vi "GetInfo.vi"(8 "error in (no error)":errorcluster, 10 "Parameter":variant, 11 "NiPxi6683H in":refnum<class "NiPxi6683H.lvclass">) -> (0 "error out":errorcluster, 2 "Info":string[](array[string]), 3 "NiPxi6683H out":refnum<class "NiPxi6683H.lvclass">)   [LabVIEW 2014, in "SyncPlugins.lvlib" / "NiPxi6683H.lvclass"]
uses:
  NiPxi6683H.lvclass
  NiPxi6682/NiPxi6682.lvclass/NiPxi6682.ctl
  NiPxi6683H.lvclass/NiPxi6683H.ctl
  NiPxi6682/Accessors/Read NiSyncHandle.vi
  Accessors/Read Triggers.vi
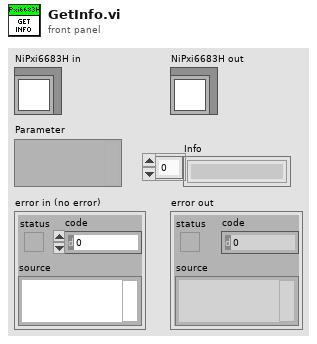
[diagram p1: front panel]
types:
  T1 = typedef "SyncPlugins.lvlib/PXI_MultiTrig.lvclass/clTrigger.ctl" = cluster{"Name":string, "DestTerm":string, "SrcTerm":string, "SyncClk":string, "Edge":i32, "Invert?":i32, "Initiated":bool, "Type":string, "TrigTime":bool}
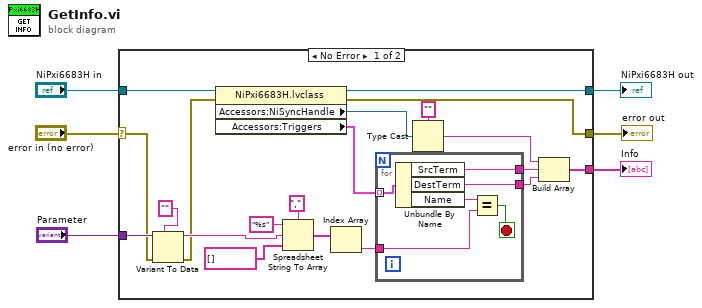
[diagram p0: block diagram]
diagram:
  n1 = case shown="No Error" "error in (no error)" {
    selector: "error in (no error)" -> [w20 w33]
    tunnel: "Parameter" -> [w25 _]
    tunnel: "NiPxi6683H in" -> [w17 w34]
    tunnel: [w16 w34] -> w3
    tunnel: [w18 w33] -> w2
    tunnel: [w9 _] -> w1
    frame No Error {
      n2 = Variant To Data(error in=w20, type="", Variant=w25) -> (data=w21:string, error out=w19:errorcluster)
      n3 = property class="NiPxi6683H.lvclass"(reference=w17, error in=w19) -> (reference out=w16:refnum<class "NiPxi6683H.lvclass">, error out=w18:errorcluster, "Accessors:NiSyncHandle"=w11:refnum<k15>, "Accessors:Triggers"=w14:T1[])
      n4 = Spreadsheet String To Array(delimiter (Tab)=",", format string="%s", spreadsheet string=w21, array type (2D Dbl)=string[] []) -> (array=w15:string[])
      n5 = Index Array(array=w15) -> (element=w13:string)  [unwired: 1 in]
      n6 = for {
        tunnel: w14 -> [w32] mode=indexing
        tunnel: w13 -> [w31]
        tunnel: [w28] -> w12
        tunnel: [w27] -> w7
        stop <- w29 stop-if-true
        n7 = Unbundle By Name(w32) -> ("SrcTerm"=w27:string, "DestTerm"=w28:string, "Name"=w30:string)
        n8 = Equal?(x=w30, y=w31) -> (x = y?=w29:bool)
      }
      n9 = Type Cast(type="", x=w11) -> (*(type *) &x=w8:string)
      n10 = Build Array(w8, w7, w12) -> (w9:string[])
    }
    frame Error {
    }
  }
  "error out" <- w2
  "NiPxi6683H out" <- w3
  "Info" <- w1
